vi "Cycle Start.vi"(8 "error in (no error)":errorcluster, 11 "Idle in":refnum<class "Idle.lvclass">) -> (0 "error out":errorcluster, 3 "Idle out":refnum<class "Idle.lvclass">)   [LabVIEW 2024, in "Idle.lvlib" / "Idle.lvclass"]
uses:
  Idle.lvclass
  Idle.lvclass/Idle.ctl
  State Pattern Actor/State Machine/State Machine/State Machine.lvclass
  C:/Program Files (x86)/National Instruments/LabVIEW 2024/vi.lib/ActorFramework/Actor/Actor.lvclass
  C:/Users/uspoaotto/OneDrive - Oregon Tool/Desktop/working copies/stateMachineActor/src/State Pattern Actor/State Machine/State Machine/State Machine.lvclass
  C:/Users/uspoaotto/OneDrive - Oregon Tool/Desktop/working copies/stateMachineActor/src/Nested State Machine Actors/Automation Controller/Automation Controller/Automation Controller.lvclass
  C:/Users/uspoaotto/OneDrive - Oregon Tool/Desktop/working copies/stateMachineActor/src/Nested State Machine Actors/Event Messages/Event Messages/Event Messages.lvclass
  C:/Users/uspoaotto/OneDrive - Oregon Tool/Desktop/working copies/stateMachineActor/src/Nested State Machine Actors/Idle/Idle/Idle.lvclass
  Active/Active/Active.lvclass
  C:/Users/uspoaotto/OneDrive - Oregon Tool/Desktop/working copies/stateMachineActor/src/Nested State Machine Actors/Active/Active/Active.lvclass
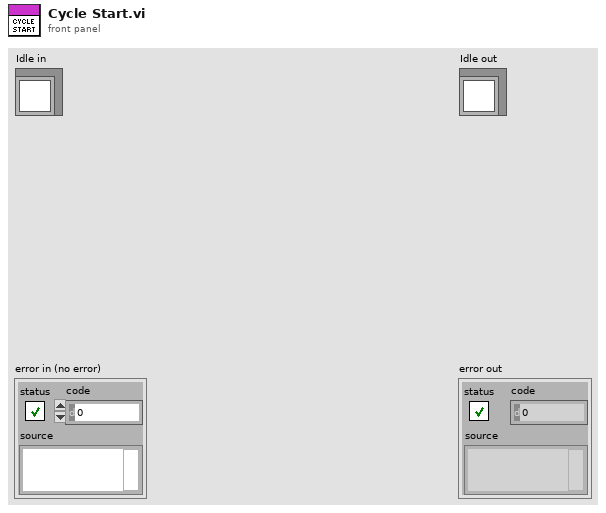
[diagram p1: front panel]
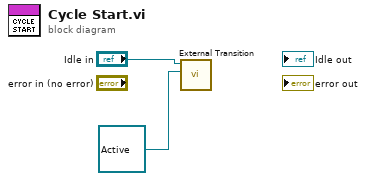
[diagram p0: block diagram]
diagram:
  n1 = call-dynamic "External Transition.vi"("Target State"=refnum<class "Active.lvclass"> refnum ("Active.lvlib:Active.lvclass"), "State Machine in"="Idle in") -> ()  [unwired: 8 in, 2 out]
